vi "main_FGV.vi"(7 "main_FGV_mods":T1, 8 "Error In":errorcluster, 11 "ParamIn":variant) -> (0 "Error Out":errorcluster, 3 "ParamOut":variant)   [LabVIEW 2016]
uses:
  main_FGV_mods.ctl
  pipe_properties.ctl
  main_FGV_data.ctl
  StressCalculations/point_data.ctl
  Ovalization/ovalization_data.ctl
  StressDist/StressDist_data.ctl
  StressDist/StressDist_single_data.ctl
  StressDist/Peirce/peirce_data.ctl
  Report/report_mods.ctl
  StressDist/StressDist_types.ctl
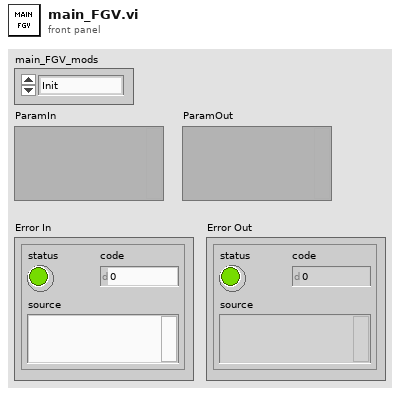
[diagram p1: front panel]
types:
  T1 = typedef "main_FGV_mods.ctl" = enum16{"Init", "PipeProps", "RSCalc", "Ovalization", "StressDist", "Peirce", "End"}
  T2 = typedef "pipe_properties.ctl" = cluster{"out_radius":dbl, "in_radius":dbl, "out_diameter":dbl, "in_diameter":dbl, "thickness":dbl, "inertia":dbl, "area":dbl}
  T3 = typedef "report_mods.ctl" = enum16{"Init", "Table", "Graph", "End"}
  T4 = typedef "main_FGV_data.ctl" = cluster{"pipe_properties":T2, "DirPath":path, "DirReport":path, "Points":T5[], "ovalization_data":T6, "StressDist_data":T7}
  T5 = typedef "point_data.ctl" = cluster{"LongStress":dbl, "CircStress":dbl, "ShearStress":dbl, "Pressure":dbl, "Angle":dbl, "Thickness":dbl, "HoleDiam":dbl}
  T6 = typedef "ovalization_data.ctl" = cluster{"AngOval":dbl[], "OvalDiam":dbl[], "Plots":cluster{"Ref":cluster{"X":dbl[], "Y":dbl[]}, "Elipse":cluster{"X":dbl[], "Y":dbl[]}, "Points":cluster{"X":dbl[], "Y":dbl[]}}, "Ampliation":dbl, "Results":cluster{"MD":dbl, "mD":dbl, "Dmed":dbl, "Oval":dbl, "ang":dbl, "X0":dbl, "Y0":dbl}}
  T7 = typedef "StressDist_data.ctl" = cluster{"Long":T8, "Circ":T8, "Shear":T8}
  T8 = typedef "StressDist_single_data.ctl" = cluster{"Plot":cluster{"Angle":dbl[], "Stress":dbl[]}[], "Fit":dbl[], "ColorMap":dbl[][], "Data":string[][], "peirce_data":T9}
  T9 = typedef "peirce_data.ctl" = cluster{"Plot":cluster{"Array":dbl[], "Array":dbl[]}[], "Index removidos":i32[]}
  T10 = typedef "StressDist_types.ctl" = enum16{"Long", "Circ", "Shear"}
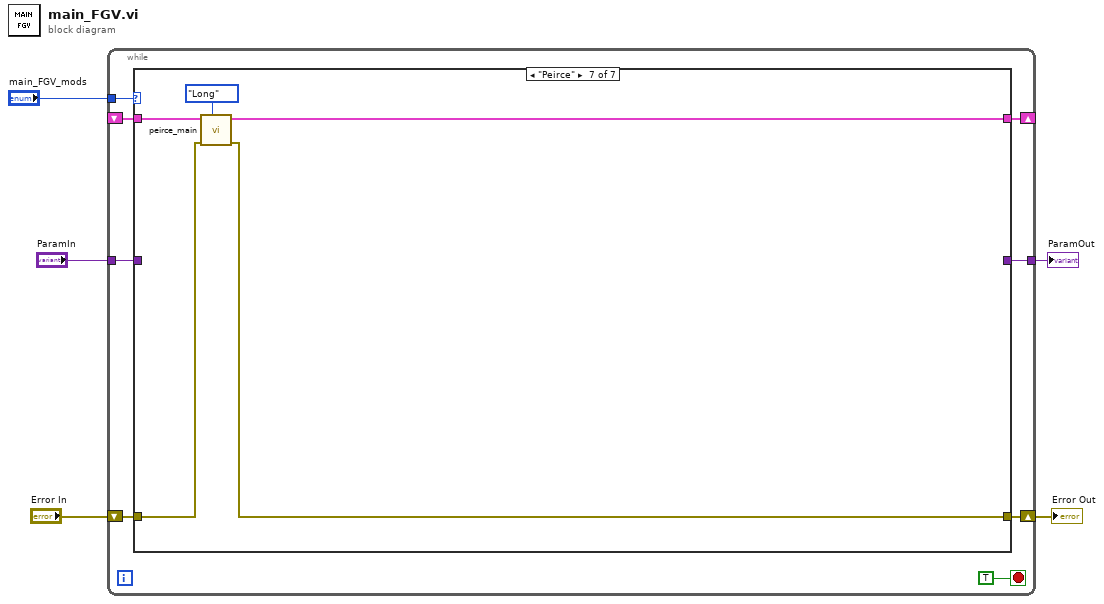
[diagram p0: block diagram]
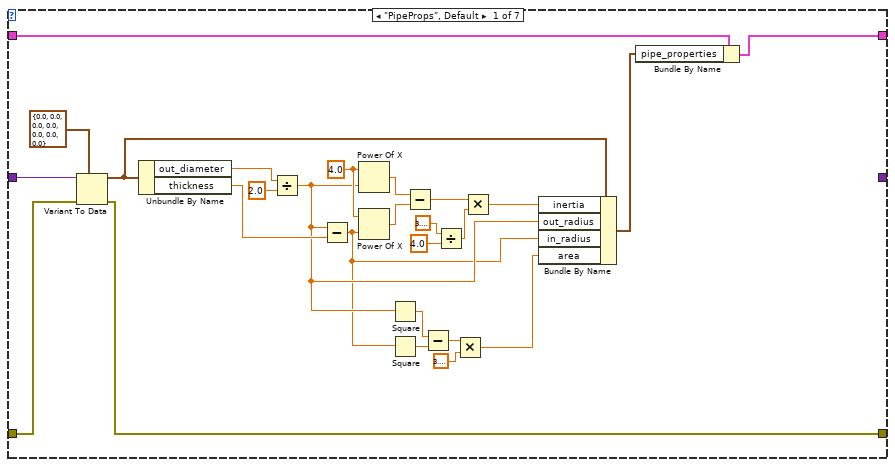
[diagram p2: hidden frame]
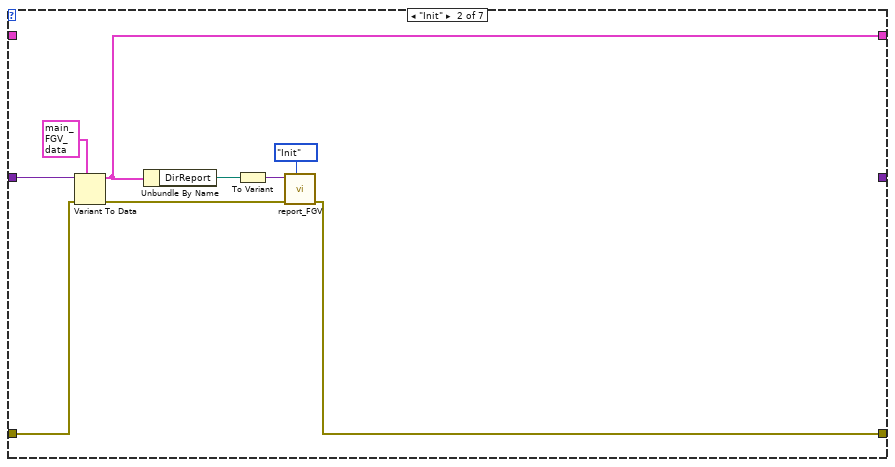
[diagram p3: hidden frame]
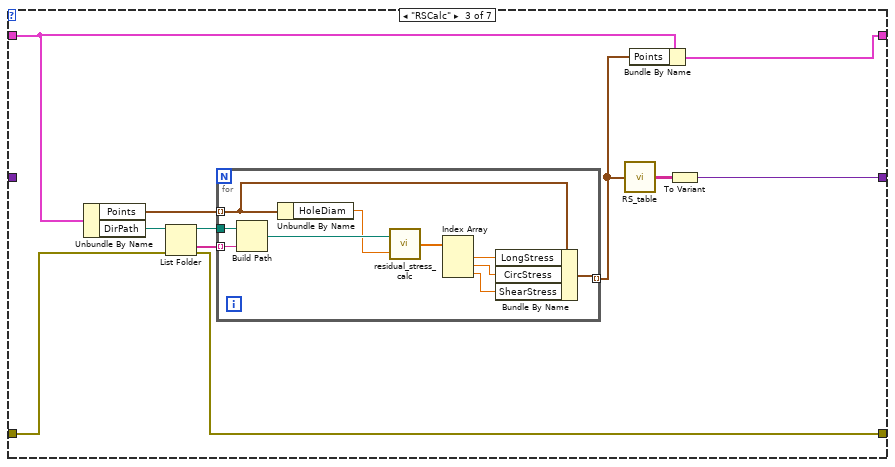
[diagram p4: hidden frame]
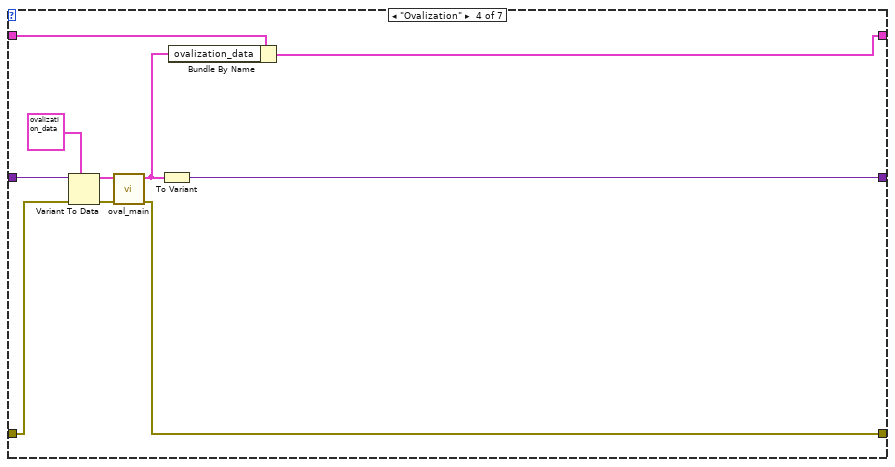
[diagram p5: hidden frame]
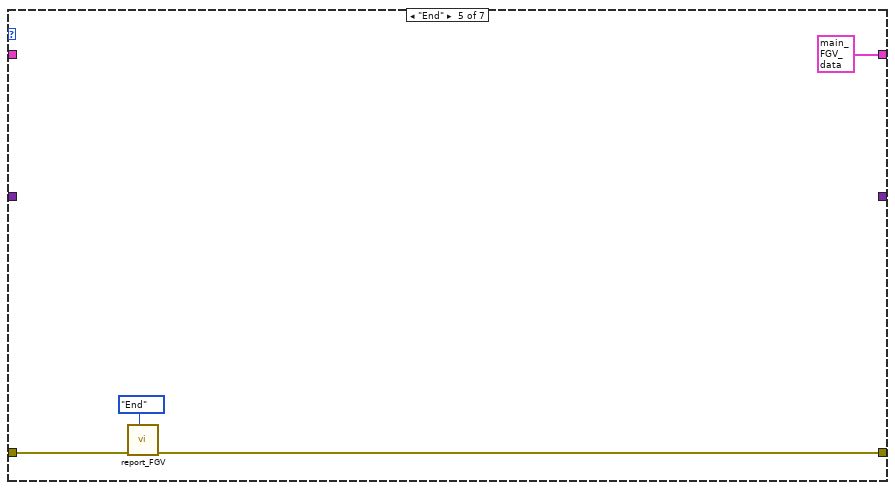
[diagram p6: hidden frame]
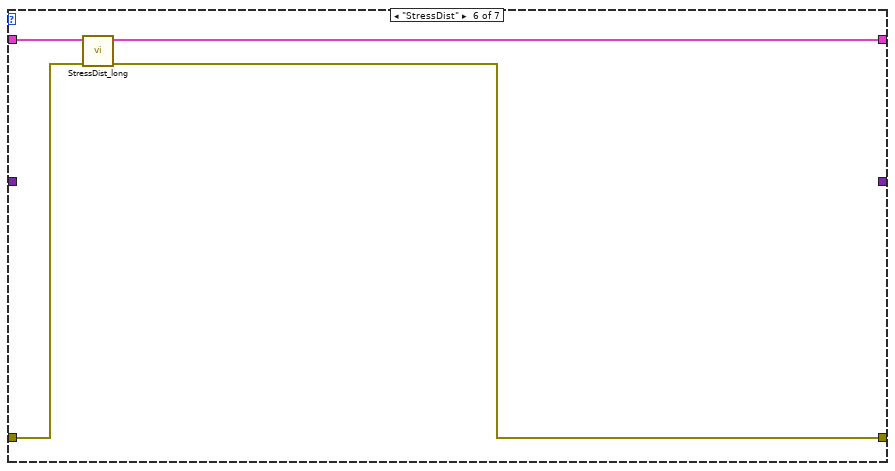
[diagram p7: hidden frame]
diagram:
  n1 = while {
    tunnel: "main_FGV_mods" -> [w12]
    tunnel: "ParamIn" -> [w11]
    shift-right: [w9] -> _
    shift-left: _ -> [w8]
    shift-right: [w7] -> w2
    shift-left: "Error In" -> [w10]
    tunnel: [w6] -> w1
    stop <- TRUE stop-if-true
    n2 = case shown="\"Peirce\"" w12 {
      tunnel: w11 -> [w39 w48 _ w79 _ _ _]
      tunnel: w10 -> [w38 w47 w59 w78 w83 w87 w91]
      tunnel: [w15 w45 w53 w73 T4 {"pipe_properties"={"out_radius"=0.0, "in_radius"=0.0, "out_diameter"=0.0, "in_diameter"=0.0, "thickness"=0.0, "inertia"=0.0, "area"=0.0}, "DirPath"=path "L:/Documentos/00 SERVIÇOS/Tensão residual/Olapa 10-2017/Dados/Primeira Seção/Furos", "DirReport"=path "L:/Documentos/00 SERVIÇOS/Tensão residual/Olapa 10-2017/RelatóriosOlapa/Teste", "Points"=[], "ovalization_data"={"AngOval"=[0.0, 60.0, 120.0, 22.5, 45.0, 67.5, 90.0, 112.5, 135.0, 157.5, 180.0], "OvalDiam"=[324.25, 324.6, 324.55, 324.25, 324.55, 324.65, 324.6, 324.65, 324.55, 324.5, 324.4], "Plots"={"Ref"={"X"=[], "Y"=[]}, "Elipse"={"X"=[], "Y"=[]}, "Points"={"X"=[], "Y"=[]}}, "Ampliation"=100.0, "Results"={"MD"=0.0, "mD"=0.0, "Dmed"=0.0, "Oval"=0.0, "ang"=0.0, "X0"=0.0, "Y0"=0.0}}, "StressDist_data"={"Long"={"Plot"=[], "Fit"=[], "ColorMap"=[], "Data"=[], "peirce_data"={"Plot"=[], "Index removidos"=[]}}, "Circ"={"Plot"=[], "Fit"=[], "ColorMap"=[], "Data"=[], "peirce_data"={"Plot"=[], "Index removidos"=[]}}, "Shear"={"Plot"=[], "Fit"=[], "ColorMap"=[], "Data"=[], "peirce_data"={"Plot"=[], "Index removidos"=[]}}}} ("main_FGV_data") w84 w89] -> w9
      tunnel: w8 -> [w17 _ w54 w74 _ w85 w92]
      tunnel: [w14 w40 w52 w75 w81 w86 w88] -> w7
      tunnel: [_ _ w51 w71 _ _ _] -> w6
      frame "PipeProps", Default {
        w27 = 4.0 ("y")
        n3 = Variant To Data(error in=w38, type=T2 {"out_radius"=0.0, "in_radius"=0.0, "out_diameter"=0.0, "in_diameter"=0.0, "thickness"=0.0, "inertia"=0.0, "area"=0.0} ("pipe_properties"), Variant=w39) -> (data=w36:T2, error out=w14:errorcluster)
        n4 = Unbundle By Name(w36) -> ("out_diameter"=w23:dbl, "thickness"=w22:dbl)
        n5 = Divide(x=w23, y=2.0) -> (x/y=w19:dbl)
        n6 = Subtract(x=w19, y=w22) -> (x-y=w18:dbl)
        n7 = Power Of X(1:w19, 2:w27) -> (0:w28:dbl)
        n8 = Power Of X(1:w18, 2:w27) -> (0:w29:dbl)
        n9 = Square(x=w19) -> (x^2=w33:dbl)
        n10 = Square(x=w18) -> (x^2=w32:dbl)
        n11 = Subtract(x=w28, y=w29) -> (x-y=w30:dbl)
        n12 = Subtract(x=w33, y=w32) -> (x-y=w34:dbl)
        n13 = Divide(x=3.141592653589793, y=4.0) -> (x/y=w31:dbl)
        n14 = Multiply(x=w34, y=3.141592653589793) -> (x*y=w20:dbl)
        n15 = Multiply(x=w30, y=w31) -> (x*y=w21:dbl)
        n16 = Bundle By Name(cluster=w36, "inertia"=w21, "out_radius"=w19, "in_radius"=w18, "area"=w20) -> (w16:T2)
        n17 = Bundle By Name(cluster=w17, "pipe_properties"=w16) -> (w15:T4)
      }
      frame "Init" {
        n18 = Variant To Data(error in=w47, type=T4 {"pipe_properties"={"out_radius"=0.0, "in_radius"=0.0, "out_diameter"=0.0, "in_diameter"=0.0, "thickness"=0.0, "inertia"=0.0, "area"=0.0}, "DirPath"=path "L:/Documentos/00 SERVIÇOS/Tensão residual/Olapa 10-2017/Dados/Primeira Seção/Furos", "DirReport"=path "L:/Documentos/00 SERVIÇOS/Tensão residual/Olapa 10-2017/RelatóriosOlapa/Teste", "Points"=[], "ovalization_data"={"AngOval"=[0.0, 60.0, 120.0, 22.5, 45.0, 67.5, 90.0, 112.5, 135.0, 157.5, 180.0], "OvalDiam"=[324.25, 324.6, 324.55, 324.25, 324.55, 324.65, 324.6, 324.65, 324.55, 324.5, 324.4], "Plots"={"Ref"={"X"=[], "Y"=[]}, "Elipse"={"X"=[], "Y"=[]}, "Points"={"X"=[], "Y"=[]}}, "Ampliation"=100.0, "Results"={"MD"=0.0, "mD"=0.0, "Dmed"=0.0, "Oval"=0.0, "ang"=0.0, "X0"=0.0, "Y0"=0.0}}, "StressDist_data"={"Long"={"Plot"=[], "Fit"=[], "ColorMap"=[], "Data"=[], "peirce_data"={"Plot"=[], "Index removidos"=[]}}, "Circ"={"Plot"=[], "Fit"=[], "ColorMap"=[], "Data"=[], "peirce_data"={"Plot"=[], "Index removidos"=[]}}, "Shear"={"Plot"=[], "Fit"=[], "ColorMap"=[], "Data"=[], "peirce_data"={"Plot"=[], "Index removidos"=[]}}}} ("main_FGV_data"), Variant=w48) -> (data=w45:T4, error out=w42:errorcluster)
        n19 = Unbundle By Name(w45) -> ("DirReport"=w44:path)
        n20 = To Variant(anything=w44) -> (Variant=w43:variant)
        n21 = call "report_FGV.vi"("report_mods"=report_mods."Init", "Error In"=w42, "Data in"=w43) -> ("Error Out"=w40:errorcluster)  [unwired: 8 in]
      }
      frame "RSCalc" {
        n22 = Unbundle By Name(w54) -> ("Points"=w55:T5[], "DirPath"=w58:path)
        n23 = List Folder(path=w58, error in=w59) -> (path out=w57:path, folder names=w56:string[], error out=w52:errorcluster)  [unwired: 2 in, 1 out]
        n24 = for {
          tunnel: w57 -> [w69]
          tunnel: w56 -> [w68] mode=indexing
          tunnel: w55 -> [w64] mode=indexing
          tunnel: [w60] -> w49 mode=indexing
          n25 = Build Path(base path=w69, name or relative path=w68) -> (appended path=w67:path)
          n26 = Unbundle By Name(w64) -> ("HoleDiam"=w66:dbl)
          n27 = call "residual_stress_calc.vi"("DiamCorrigido"=w66, "Pasta do ensaio"=w67) -> ("ResultsDist"=w65:dbl[])
          n28 = Index Array(array=w65) -> (element #1=w63:dbl, element #2=w62:dbl, element #3=w61:dbl)  [unwired: 3 in]
          n29 = Bundle By Name(cluster=w64, "LongStress"=w63, "CircStress"=w62, "ShearStress"=w61) -> (w60:T5)
        }
        n30 = call "RS_table.vi"("RSpoints"=w49) -> ("Table"=w50:string[][])
        n31 = Bundle By Name(cluster=w54, "Points"=w49) -> (w53:T4)
        n32 = To Variant(anything=w50) -> (Variant=w51:variant)
      }
      frame "Ovalization" {
        n33 = Variant To Data(error in=w78, type=T6 {"AngOval"=[0.0, 60.0, 120.0, 22.5, 45.0, 67.5, 90.0, 112.5, 135.0, 157.5, 180.0], "OvalDiam"=[324.25, 324.6, 324.55, 324.25, 324.55, 324.65, 324.6, 324.65, 324.55, 324.5, 324.4], "Plots"={"Ref"={"X"=[], "Y"=[]}, "Elipse"={"X"=[], "Y"=[]}, "Points"={"X"=[], "Y"=[]}}, "Ampliation"=100.0, "Results"={"MD"=0.0, "mD"=0.0, "Dmed"=0.0, "Oval"=0.0, "ang"=0.0, "X0"=0.0, "Y0"=0.0}} ("ovalization_data"), Variant=w79) -> (data=w76:T6, error out=w77:errorcluster)
        n34 = call "oval_main.vi"("Error In"=w77, "ovalization_data"=w76) -> ("Error Out"=w75:errorcluster, "output ovalization_data-out"=w72:T6)  [unwired: 8 in]
        n35 = To Variant(anything=w72) -> (Variant=w71:variant)
        n36 = Bundle By Name(cluster=w74, "ovalization_data"=w72) -> (w73:T4)
      }
      frame "End" {
        n37 = call "report_FGV.vi"("report_mods"=report_mods."End", "Error In"=w83) -> ("Error Out"=w81:errorcluster)  [unwired: 9 in]
      }
      frame "StressDist" {
        n38 = call "StressDist_long.vi"("Error In"=w87, "main_FGV_data"=w85) -> ("Error Out"=w86:errorcluster, "main_FGV_data-out"=w84:T4)  [unwired: 8 in]
      }
      frame "Peirce" {
        n39 = call "peirce_main.vi"("StressDist_types"=StressDist_types."Long", "Error In"=w91, "main_FGV_data"=w92) -> ("Error Out"=w88:errorcluster, "main_FGV_data-out"=w89:T4)  [unwired: 7 in]
      }
    }
  }
  "ParamOut" <- w1
  "Error Out" <- w2
